vi "Example Simple.vi"() -> ()   [LabVIEW 2013]
uses:
  C:/tf/play/labview/Tinkerforge.dll
  Tinkerforge.dll
panel:
  out "count":i32
  in  "uid":string="8e7"
  in  "port":i32=4223
  in  "host":string="localhost"
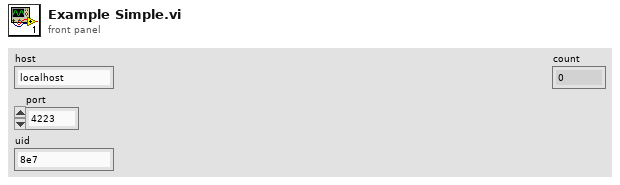
[diagram p1: front panel]
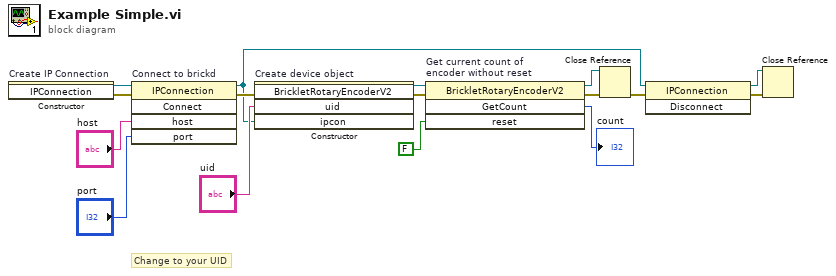
[diagram p0: block diagram]
diagram:
  # "Change to your UID"
  n1 = constructor on="Create IP Connection" class="IPConnection"() -> (reference out=w16:refnum<k24>, error out=w3:errorcluster)  [unwired: 3 in, 1 out]
  n2 = invoke on="Connect to brickd" class="IPConnection" method="Connect"(reference=w16, error in=w3, "host"="host", "port"="port") -> (reference out=w5:refnum<k24>, error out=w12:errorcluster)  [unwired: 1 in, 3 out]
  n3 = constructor on="Create device object" class="BrickletRotaryEncoderV2"(error in=w12, "uid"="uid", "ipcon"=w5) -> (reference out=w10:refnum<k24>, error out=w11:errorcluster)  [unwired: 2 in, 3 out]
  n4 = invoke on="Get current count of\nencoder without reset" class="BrickletRotaryEncoderV2" method="GetCount"(reference=w10, error in=w11, "reset"=FALSE) -> (reference out=w8:refnum<k24>, error out=w9:errorcluster, "GetCount"=→"count":i32)  [unwired: 1 in, 1 out]
  n5 = Close Reference(reference=w8, error in (no error)=w9) -> (error out=w7:errorcluster)
  n6 = invoke class="IPConnection" method="Disconnect"(reference=w5, error in=w7) -> (reference out=w4:refnum<k24>, error out=w6:errorcluster)  [unwired: 1 in, 1 out]
  n7 = Close Reference(reference=w4, error in (no error)=w6) -> ()  [unwired: 1 out]
